vi "TestBiocuiniqueTimer_Alpha 6.vi"() -> ()   [LabVIEW 2021]
uses:
  <vilib>/Utility/NIReport.llb/Report Type.ctl
  <extravilib>/ChannelInstances/Tag-u8/Read With Abort.vi
  <extravilib>/ChannelInstances/Tag-bool/Read With Abort.vi
  <extravilib>/ChannelInstances/Tag-bool/Write With Abort.vi
  <extravilib>/ChannelInstances/Tag-u8/Write With Abort.vi
  <extravilib>/ChannelInstances/Tag-u8/Instantiate.vi
  <extravilib>/ChannelInstances/Tag-bool/Instantiate.vi
  <extravilib>/ChannelInstances/Tag-u8/EndpointRead.vi
  <vilib>/addons/_office/excel.llb/Excel Easy Table (str).vi
  <extravilib>/ChannelInstances/Tag-bool/EndpointRead.vi
  <extravilib>/ChannelInstances/Tag-bool/Endpoint.vi
  <extravilib>/ChannelInstances/Tag-u8/Endpoint.vi
  <vilib>/Utility/NIReport.llb/NI_report.lvclass
  <vilib>/LabVIEW Interface for Arduino/LabVIEW Interface for Arduino.lvlib
  <vilib>/Utility/NIReport.llb/NI_ReportGenerationCore.lvlib
  <vilib>/addons/_office/NI_ReportGenerationToolkit.lvlib
  <vilib>/Utility/NIReport.llb/Excel/NI_Excel.lvclass
  <extravilib>/ChannelInstances/Tag-bool.lvlib
  <extravilib>/ChannelInstances/Tag-u8.lvlib
panel:
  out "CONTADOR":dbl
  in  "2 minutos cada 2 horas  de 7am a 8pm":path
  out "BOMBA 2":bool
  out "BOMBA 1":bool
  out "VÁLVULA 4":bool
  out "VÁLVULA 3":bool
  out "VÁLVULA 2":bool
  out "VÁLVULA 1":bool
  in  "VISA resource":refnum<visa-resource-name>
  in  "stop":bool
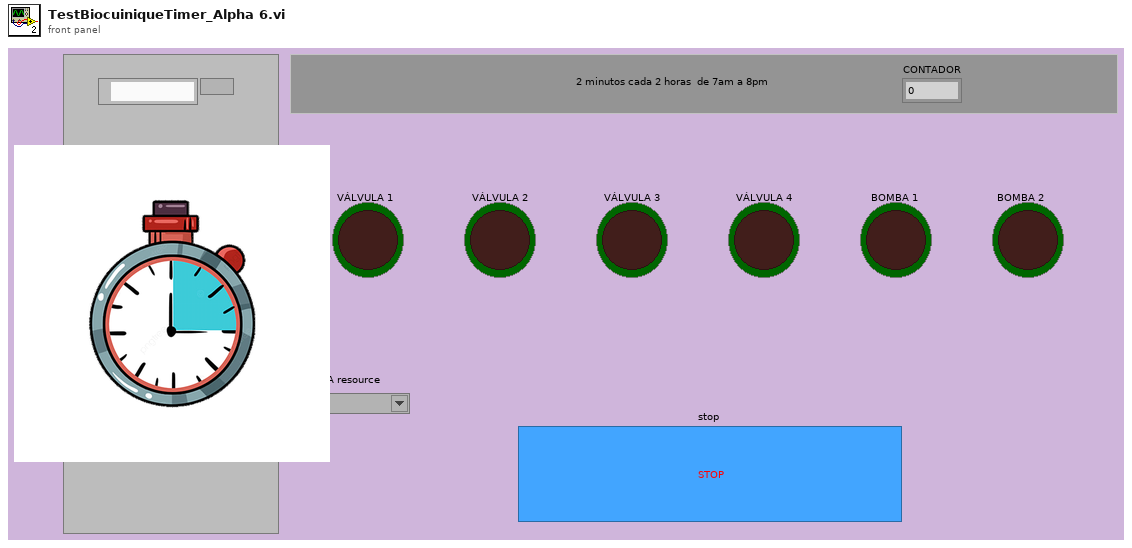
[diagram p1: front panel]
types:
  T1 = typedef "NI_ReportGenerationCore.lvlib/Report Type.ctl" = enum16{"HTML", "Word", "Excel"}
  T2 = typedef "LabVIEW Interface for Arduino.lvlib/Arduino Resource.ctl" = cluster{"VISA resource":refnum<visa-resource-name>, "Board Type":T3, "Connection Type":enum8{"USB / Serial"}, "Bytes Per Packet (15)":u8}
  T3 = typedef "LabVIEW Interface for Arduino.lvlib/Board Type.ctl" = enum16{"Uno", "Dimuelanove w/Atmega 328", "Mega 2560"}
  T4 = typedef "Tag-u8.lvlib/))Channel.ctl" = refnum<queue>
  T5 = typedef "Tag-bool.lvlib/))Channel.ctl" = refnum<queue>
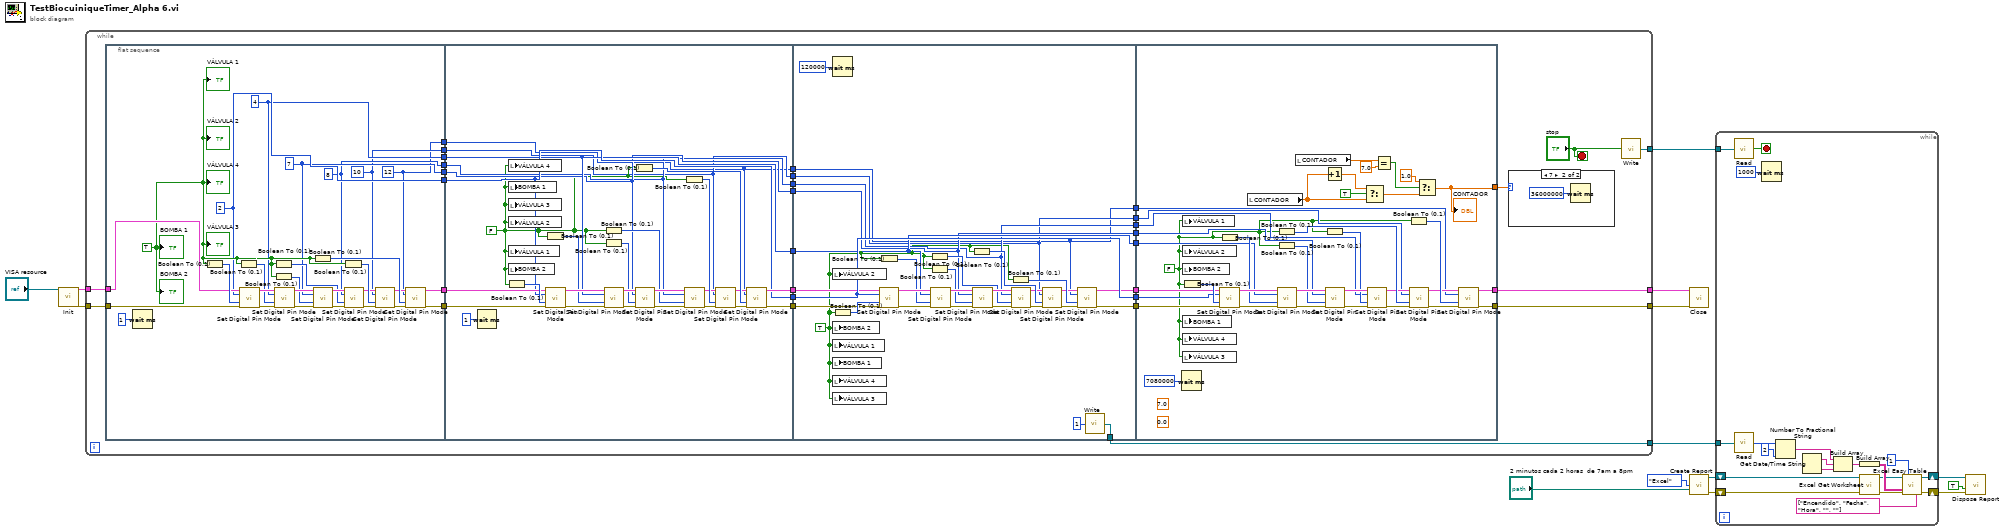
[diagram p0: block diagram]
diagram:
  n1 = call <vilib>:"Init.vi"("VISA resource"="VISA resource") -> ("Arduino Resource"=w11:T2, "error out"=w10:errorcluster)  [unwired: 17 in]
  n2 = while {
    tunnel: w11 -> [w20]
    tunnel: w10 -> [w19]
    tunnel: [w22] -> w13
    tunnel: [w21] -> w12
    tunnel: [w18] -> w1
    tunnel: [w16] -> w2
    stop <- "stop" stop-if-true
    n3 = flat-sequence {
      tunnel: w20 -> [w73]
      tunnel: [w62] -> w46
      tunnel: w19 -> [w61]
      tunnel: [w55] -> w45
      tunnel: [w53] -> w44
      tunnel: [w52] -> w43
      tunnel: [w51] -> w42
      tunnel: [w50] -> w41
      tunnel: [w49] -> w40
      tunnel: [w48] -> w39
      tunnel: w46 -> [w92]
      tunnel: w45 -> [w90]
      tunnel: w44 -> [w82]
      tunnel: w43 -> [w81]
      tunnel: w42 -> [w80]
      tunnel: w41 -> [w79]
      tunnel: w40 -> [w78]
      tunnel: w39 -> [w77]
      tunnel: [w91] -> w38
      tunnel: [w83] -> w37
      tunnel: [w82] -> w36
      tunnel: [w81] -> w35
      tunnel: [w80] -> w34
      tunnel: [w79] -> w33
      tunnel: [w78] -> w32
      tunnel: [w77] -> w31
      tunnel: w38 -> [w109]
      tunnel: w37 -> [w110]
      tunnel: w36 -> [w116]
      tunnel: w35 -> [w115]
      tunnel: w34 -> [w114]
      tunnel: w33 -> [w113]
      tunnel: w32 -> [w112]
      tunnel: w31 -> [w111]
      tunnel: [w116] -> w30
      tunnel: [w115] -> w29
      tunnel: [w114] -> w28
      tunnel: [w113] -> w27
      tunnel: [w112] -> w26
      tunnel: [w111] -> w25
      tunnel: [w108] -> w24
      tunnel: [w107] -> w23
      tunnel: [w104] -> w18
      tunnel: w30 -> [w154]
      tunnel: w29 -> [w153]
      tunnel: w28 -> [w152]
      tunnel: w27 -> [w151]
      tunnel: w26 -> [w150]
      tunnel: w25 -> [w149]
      tunnel: w24 -> [w148]
      tunnel: w23 -> [w147]
      tunnel: [w146] -> w22
      tunnel: [w145] -> w21
      tunnel: [w134] -> w15
      frame #0 {
        w48 = u8 12 ("BOMBA 2")
        w49 = u8 10 ("BOMBA 1")
        w50 = u8 8 ("VALVULA 4")
        w51 = u8 7 ("VALVULA 3")
        w52 = u8 4 ("VALVULA 2")
        w53 = u8 2 ("VALVULA 1")
        w54 = TRUE
        n4 = Wait (ms)(milliseconds to wait=u32 1) -> ()  [unwired: 1 out]
        n5 = Boolean To (0,1)(Boolean=w54) -> (0, 1=w75:i16)
        n6 = Boolean To (0,1)(Boolean=w54) -> (0, 1=w69:i16)
        n7 = call <vilib>:"Set Digital Pin Mode.vi"("Arduino Resource"=w73, "Digital I/O Pin"=w53, "Pin Mode (Input)"=w75, "error in"=w61) -> ("Arduino Resource"=w72:T2, "error out"=w60:errorcluster)  [unwired: 10 in]
        n8 = Boolean To (0,1)(Boolean=w54) -> (0, 1=w67:i16)
        n9 = Boolean To (0,1)(Boolean=w54) -> (0, 1=w68:i16)
        n10 = call <vilib>:"Set Digital Pin Mode.vi"("Arduino Resource"=w72, "Digital I/O Pin"=w52, "Pin Mode (Input)"=w69, "error in"=w60) -> ("Arduino Resource"=w71:T2, "error out"=w59:errorcluster)  [unwired: 10 in]
        n11 = Boolean To (0,1)(Boolean=w54) -> (0, 1=w66:i16)
        n12 = call <vilib>:"Set Digital Pin Mode.vi"("Arduino Resource"=w71, "Digital I/O Pin"=w51, "Pin Mode (Input)"=w68, "error in"=w59) -> ("Arduino Resource"=w70:T2, "error out"=w58:errorcluster)  [unwired: 10 in]
        n13 = Boolean To (0,1)(Boolean=w54) -> (0, 1=w65:i16)
        n14 = call <vilib>:"Set Digital Pin Mode.vi"("Arduino Resource"=w70, "Digital I/O Pin"=w50, "Pin Mode (Input)"=w67, "error in"=w58) -> ("Arduino Resource"=w64:T2, "error out"=w57:errorcluster)  [unwired: 10 in]
        n15 = call <vilib>:"Set Digital Pin Mode.vi"("Arduino Resource"=w64, "Digital I/O Pin"=w49, "Pin Mode (Input)"=w65, "error in"=w57) -> ("Arduino Resource"=w63:T2, "error out"=w56:errorcluster)  [unwired: 10 in]
        n16 = call <vilib>:"Set Digital Pin Mode.vi"("Arduino Resource"=w63, "Digital I/O Pin"=w48, "Pin Mode (Input)"=w66, "error in"=w56) -> ("Arduino Resource"=w62:T2, "error out"=w55:errorcluster)  [unwired: 10 in]
        "VÁLVULA 1" <- w54
        "VÁLVULA 2" <- w54
        "VÁLVULA 3" <- w54
        "VÁLVULA 4" <- w54
        "BOMBA 1" <- w54
        "BOMBA 2" <- w54
      }
      frame #1 {
        w76 = FALSE
        n17 = Wait (ms)(milliseconds to wait=u32 1) -> ()  [unwired: 1 out]
        n18 = Boolean To (0,1)(Boolean=w76) -> (0, 1=w102:i16)
        n19 = local write "VÁLVULA 4"(w76) -> ()
        n20 = local write "BOMBA 1"(w76) -> ()
        n21 = local write "VÁLVULA 3"(w76) -> ()
        n22 = local write "VÁLVULA 2"(w76) -> ()
        n23 = local write "VÁLVULA 1"(w76) -> ()
        n24 = local write "BOMBA 2"(w76) -> ()
        n25 = Boolean To (0,1)(Boolean=w76) -> (0, 1=w98:i16)
        n26 = call <vilib>:"Set Digital Pin Mode.vi"("Arduino Resource"=w92, "Digital I/O Pin"=w82, "Pin Mode (Input)"=w102, "error in"=w90) -> ("Arduino Resource"=w101:T2, "error out"=w89:errorcluster)  [unwired: 10 in]
        n27 = Boolean To (0,1)(Boolean=w76) -> (0, 1=w86:i16)
        n28 = Boolean To (0,1)(Boolean=w76) -> (0, 1=w97:i16)
        n29 = call <vilib>:"Set Digital Pin Mode.vi"("Arduino Resource"=w101, "Digital I/O Pin"=w81, "Pin Mode (Input)"=w98, "error in"=w89) -> ("Arduino Resource"=w100:T2, "error out"=w88:errorcluster)  [unwired: 10 in]
        n30 = Boolean To (0,1)(Boolean=w76) -> (0, 1=w96:i16)
        n31 = call <vilib>:"Set Digital Pin Mode.vi"("Arduino Resource"=w100, "Digital I/O Pin"=w80, "Pin Mode (Input)"=w97, "error in"=w88) -> ("Arduino Resource"=w99:T2, "error out"=w87:errorcluster)  [unwired: 10 in]
        n32 = Boolean To (0,1)(Boolean=w76) -> (0, 1=w95:i16)
        n33 = call <vilib>:"Set Digital Pin Mode.vi"("Arduino Resource"=w99, "Digital I/O Pin"=w79, "Pin Mode (Input)"=w86, "error in"=w87) -> ("Arduino Resource"=w94:T2, "error out"=w85:errorcluster)  [unwired: 10 in]
        n34 = call <vilib>:"Set Digital Pin Mode.vi"("Arduino Resource"=w94, "Digital I/O Pin"=w78, "Pin Mode (Input)"=w95, "error in"=w85) -> ("Arduino Resource"=w93:T2, "error out"=w84:errorcluster)  [unwired: 10 in]
        n35 = call <vilib>:"Set Digital Pin Mode.vi"("Arduino Resource"=w93, "Digital I/O Pin"=w77, "Pin Mode (Input)"=w96, "error in"=w84) -> ("Arduino Resource"=w91:T2, "error out"=w83:errorcluster)  [unwired: 10 in]
      }
      frame #2 {
        w106 = TRUE
        n36 = Wait (ms)(milliseconds to wait=u32 120000) -> ()  [unwired: 1 out]
        n37 = local write "VÁLVULA 2"(w106) -> ()
        n38 = Boolean To (0,1)(Boolean=w106) -> (0, 1=w133:i16)
        n39 = local write "BOMBA 2"(w106) -> ()
        n40 = local write "VÁLVULA 1"(w106) -> ()
        n41 = local write "BOMBA 1"(w106) -> ()
        n42 = local write "VÁLVULA 4"(w106) -> ()
        n43 = local write "VÁLVULA 3"(w106) -> ()
        n44 = Boolean To (0,1)(Boolean=w106) -> (0, 1=w128:i16)
        n45 = call <vilib>:"Set Digital Pin Mode.vi"("Arduino Resource"=w109, "Digital I/O Pin"=w116, "Pin Mode (Input)"=w133, "error in"=w110) -> ("Arduino Resource"=w131:T2, "error out"=w121:errorcluster)  [unwired: 10 in]
        n46 = Boolean To (0,1)(Boolean=w106) -> (0, 1=w126:i16)
        n47 = Boolean To (0,1)(Boolean=w106) -> (0, 1=w127:i16)
        n48 = call <vilib>:"Set Digital Pin Mode.vi"("Arduino Resource"=w131, "Digital I/O Pin"=w115, "Pin Mode (Input)"=w128, "error in"=w121) -> ("Arduino Resource"=w130:T2, "error out"=w120:errorcluster)  [unwired: 10 in]
        n49 = Boolean To (0,1)(Boolean=w106) -> (0, 1=w124:i16)
        n50 = call <vilib>:"Set Digital Pin Mode.vi"("Arduino Resource"=w130, "Digital I/O Pin"=w114, "Pin Mode (Input)"=w127, "error in"=w120) -> ("Arduino Resource"=w129:T2, "error out"=w119:errorcluster)  [unwired: 10 in]
        n51 = Boolean To (0,1)(Boolean=w106) -> (0, 1=w125:i16)
        n52 = call <vilib>:"Set Digital Pin Mode.vi"("Arduino Resource"=w129, "Digital I/O Pin"=w113, "Pin Mode (Input)"=w126, "error in"=w119) -> ("Arduino Resource"=w123:T2, "error out"=w118:errorcluster)  [unwired: 10 in]
        n53 = call <vilib>:"Set Digital Pin Mode.vi"("Arduino Resource"=w123, "Digital I/O Pin"=w112, "Pin Mode (Input)"=w124, "error in"=w118) -> ("Arduino Resource"=w122:T2, "error out"=w117:errorcluster)  [unwired: 10 in]
        n54 = call <vilib>:"Set Digital Pin Mode.vi"("Arduino Resource"=w122, "Digital I/O Pin"=w111, "Pin Mode (Input)"=w125, "error in"=w117) -> ("Arduino Resource"=w108:T2, "error out"=w107:errorcluster)  [unwired: 10 in]
        n55 = call <extravilib>:"Write.vi"("element"=u8 1 ("Digital I/O Pin")) -> ("channel"=w104:T4)  [unwired: 1 out]
      }
      frame #3 {
        (unwired) 0.0 ("CONTADOR")
        (unwired) 7.0 ("y")
        w144 = FALSE
        n56 = Wait (ms)(milliseconds to wait=u32 7080000) -> ()  [unwired: 1 out]
        n57 = local write "VÁLVULA 1"(w144) -> ()
        n58 = local write "VÁLVULA 2"(w144) -> ()
        n59 = local write "BOMBA 2"(w144) -> ()
        n60 = Boolean To (0,1)(Boolean=w144) -> (0, 1=w170:i16)
        n61 = local write "BOMBA 1"(w144) -> ()
        n62 = local write "VÁLVULA 4"(w144) -> ()
        n63 = local write "VÁLVULA 3"(w144) -> ()
        n64 = Boolean To (0,1)(Boolean=w144) -> (0, 1=w166:i16)
        n65 = call <vilib>:"Set Digital Pin Mode.vi"("Arduino Resource"=w148, "Digital I/O Pin"=w154, "Pin Mode (Input)"=w170, "error in"=w147) -> ("Arduino Resource"=w169:T2, "error out"=w159:errorcluster)  [unwired: 10 in]
        n66 = local read "CONTADOR"() -> (w140:dbl)
        n67 = Boolean To (0,1)(Boolean=w144) -> (0, 1=w162:i16)
        n68 = Boolean To (0,1)(Boolean=w144) -> (0, 1=w165:i16)
        n69 = call <vilib>:"Set Digital Pin Mode.vi"("Arduino Resource"=w169, "Digital I/O Pin"=w153, "Pin Mode (Input)"=w166, "error in"=w159) -> ("Arduino Resource"=w168:T2, "error out"=w158:errorcluster)  [unwired: 10 in]
        n70 = local read "CONTADOR"() -> (w138:dbl)
        n71 = Increment(x=w140) -> (x+1=w141:dbl)
        n72 = Boolean To (0,1)(Boolean=w144) -> (0, 1=w164:i16)
        n73 = call <vilib>:"Set Digital Pin Mode.vi"("Arduino Resource"=w168, "Digital I/O Pin"=w152, "Pin Mode (Input)"=w165, "error in"=w158) -> ("Arduino Resource"=w167:T2, "error out"=w157:errorcluster)  [unwired: 10 in]
        n74 = Select(t=w141, s=TRUE, f=w140) -> (s? t:f=w142:dbl)
        n75 = call <vilib>:"Set Digital Pin Mode.vi"("Arduino Resource"=w167, "Digital I/O Pin"=w151, "Pin Mode (Input)"=w164, "error in"=w157) -> ("Arduino Resource"=w161:T2, "error out"=w156:errorcluster)  [unwired: 10 in]
        n76 = Equal?(x=w138, y=7.0) -> (x = y?=w136:bool)
        n77 = Boolean To (0,1)(Boolean=w144) -> (0, 1=w163:i16)
        n78 = call <vilib>:"Set Digital Pin Mode.vi"("Arduino Resource"=w161, "Digital I/O Pin"=w150, "Pin Mode (Input)"=w162, "error in"=w156) -> ("Arduino Resource"=w160:T2, "error out"=w155:errorcluster)  [unwired: 10 in]
        n79 = Select(t=1.0, s=w136, f=w142) -> (s? t:f=w134:dbl)
        "CONTADOR" <- w134
        n80 = call <vilib>:"Set Digital Pin Mode.vi"("Arduino Resource"=w160, "Digital I/O Pin"=w149, "Pin Mode (Input)"=w163, "error in"=w155) -> ("Arduino Resource"=w146:T2, "error out"=w145:errorcluster)  [unwired: 10 in]
      }
    }
    n81 = case shown="7" w15 {
      frame 0, Default {
      }
      frame 7 {
        n82 = Wait (ms)(milliseconds to wait=u32 36000000) -> ()  [unwired: 1 out]
      }
    }
    n83 = call <extravilib>:"Write.vi"("element"="stop") -> ("channel"=w16:T5)  [unwired: 1 out]
  }
  n84 = call <vilib>:"Close.vi"("Arduino Resource"=w13, "error in"=w12) -> ()  [unwired: 13 in, 1 out]
  n85 = call <vilib>:"Create Report.vi"("report type"=Report_Type."Excel", "template (empty)"="2 minutos cada 2 horas  de 7am a 8pm") -> ("report out"=w6:refnum<class "NI_report.lvclass">, "error out"=w7:errorcluster)  [unwired: 12 in]
  n86 = while {
    shift-right: [w180] -> w4
    shift-left: w7 -> [w185]
    shift-right: [w181] -> w5
    shift-left: w6 -> [w183]
    tunnel: w2 -> [w176]
    tunnel: w1 -> [w171]
    stop <- w175 stop-if-true
    n87 = call <extravilib>:"Read.vi"("channel"=w176) -> ("element"=w175:bool)  [unwired: 1 in, 1 out]
    n88 = call <extravilib>:"Read.vi"("channel"=w171) -> ("element"=w173:u8)  [unwired: 1 in, 1 out]
    n89 = Wait (ms)(milliseconds to wait=u32 1000) -> ()  [unwired: 1 out]
    n90 = Number To Fractional String(number=w173, precision (6)=i16 2) -> (F-format string=w172:string)  [unwired: 2 in]
    n91 = Get Date/Time String() -> (date string=w189:string, time string=w188:string)  [unwired: 3 in]
    n92 = Build Array(w172, w189, w188) -> (w187:string[])
    n93 = Build Array(w187) -> (w186:string[][])
    n94 = call <vilib>:"Excel Get Worksheet.vi"("report in"=w183, "error in (no error)"=w185) -> ("report out"=w182:refnum<class "NI_report.lvclass">, "error out"=w184:errorcluster)  [unwired: 12 in]
    n95 = call-poly <vilib>:"Excel Easy Table.vi"("report in"=w182, "iteration"=1, "text data"=w186, "error in (no error)"=w184, "column headers"=string[] ["Encendido", "Fecha", "Hora", "", ""]) -> ("report out"=w181:refnum<class "NI_report.lvclass">, "error out"=w180:errorcluster)  [unwired: 6 in, 3 out]
  }
  n96 = call-dynamic "Dispose Report.vi"("report in"=w5, "save changes? (F)"=TRUE, "error in (no error)"=w4) -> ()  [unwired: 12 in, 1 out]
